vi "lab_3.vi"() -> ()   [LabVIEW 2025]
uses:
  Labview-master/Lab_3/HR_Data_Structure.ctl
  Labview-master/Lab_3/Raw_Data_IN_HR.ctl
  Labview-master/Lab_3/Runner_Data_Structure.ctl
panel:
  out "XY Graph":T1(graph)
  out "BPM":cluster{"Time":timestamp[], "Bpm":i32[]}(graph)
  out "HEART RATE ZONE":string[][](array[string])
  out "error out":errorcluster
  in  "error in":errorcluster
  in  "File Path (dialog if empty)":path
  in  "Runner's Data":T2
  in  "HR Data Structure":T3 {"Raw Data"."Time" format="%<%x %.3X>T"}
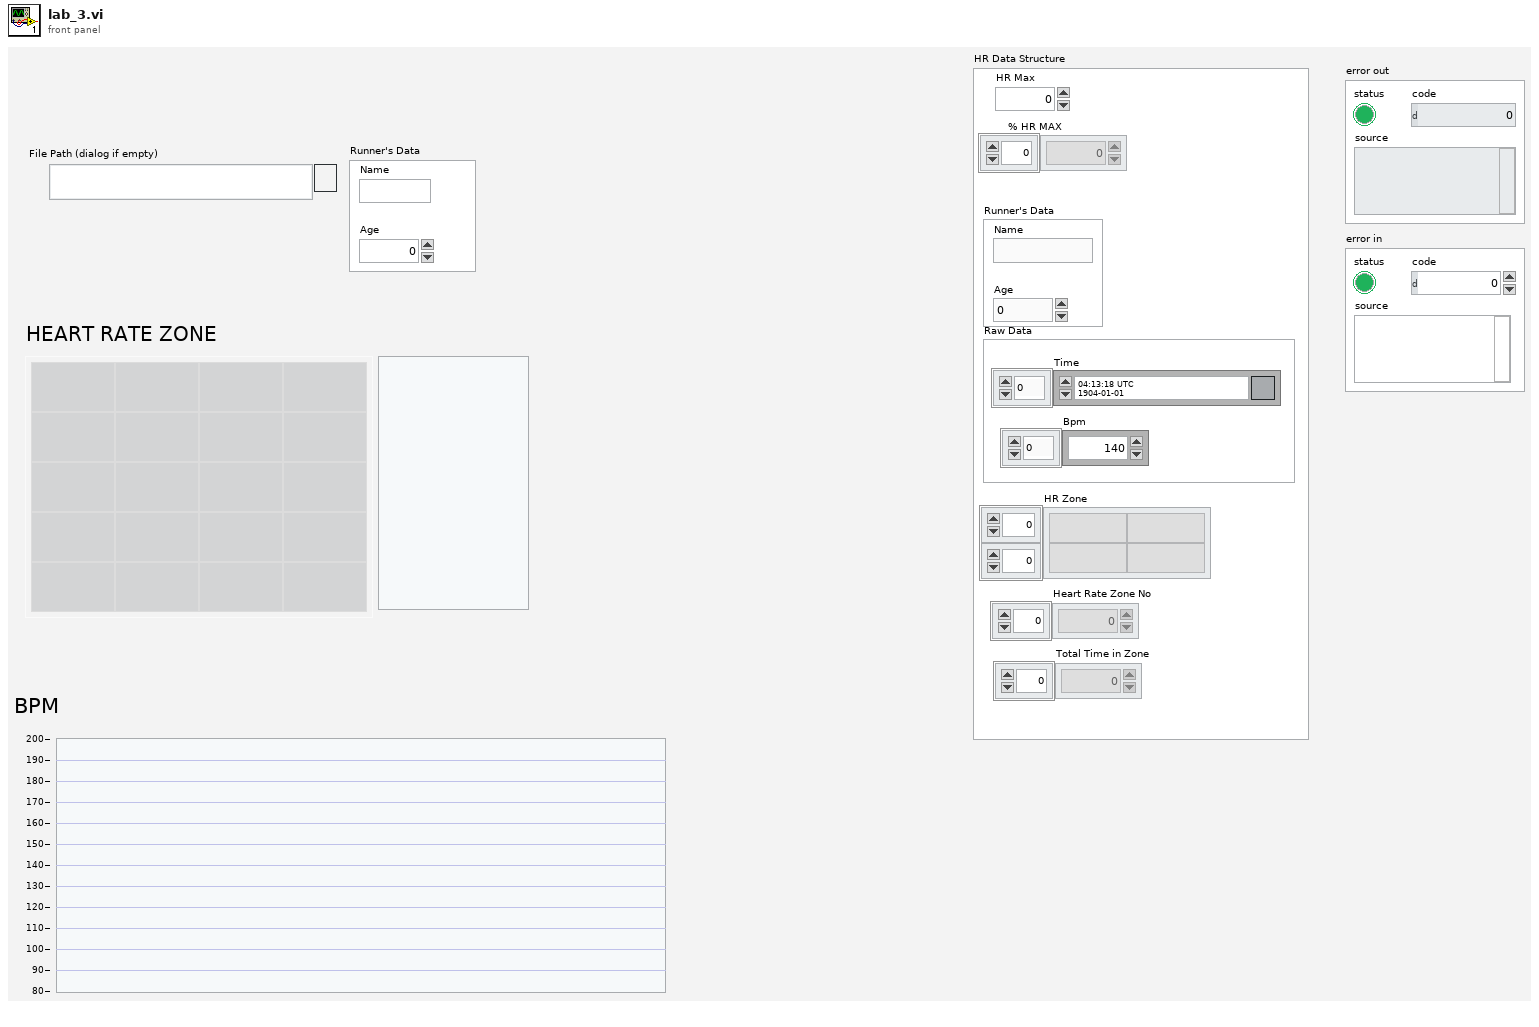
[diagram p1: front panel]
types:
  T1 = cluster{"Total Time in Zone":dbl[], "Heart Rate Zone No":dbl[]}
  T2 = typedef "Runner_Data_Structure.ctl" = cluster{"Name":string, "Age":i32}
  T3 = typedef "HR_Data_Structure.ctl" = cluster{"HR Max":i32, "% HR MAX ":dbl[], "Raw Data":T4, "Runner's Data":T2, "HR Zone":string[][], "Total Time in Zone":dbl[], "Heart Rate Zone No":dbl[]}
  T4 = typedef "Raw_Data_IN_HR.ctl" = cluster{"Time":timestamp[], "Bpm":i32[]}
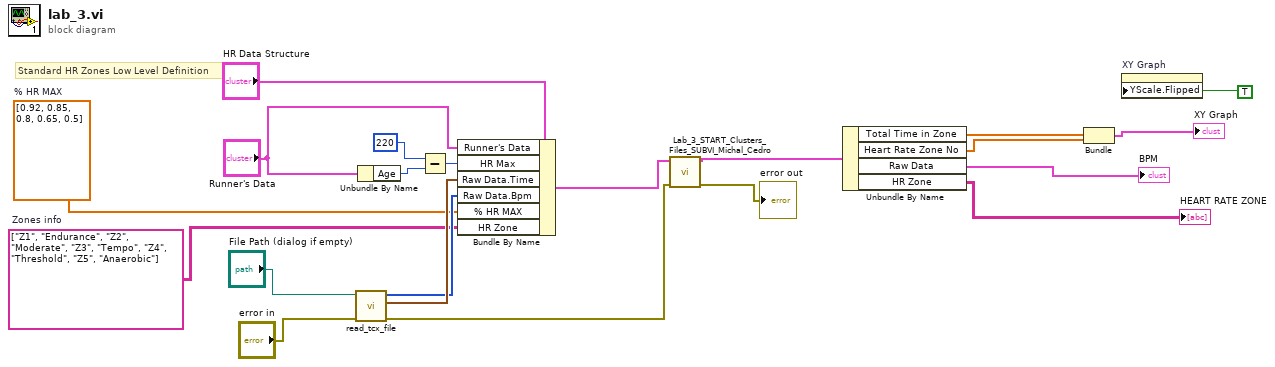
[diagram p0: block diagram]
diagram:
  w8 = string[][] [["Z1", "Endurance"], ["Z2", "Moderate"], ["Z3", "Tempo"], ["Z4", "Threshold"], ["Z5", "Anaerobic"]]  # Zones info
  w9 = dbl[] [0.92, 0.85, 0.8, 0.65, 0.5]  # % HR MAX
  # "Standard HR Zones Low Level Definition"
  n1 = call "read_tcx_file.vi"("error in"="error in", "File Path"="File Path (dialog if empty)") -> ("error out"=w1:errorcluster, "Time"=w14:timestamp[], "Bpm"=w12:i32[])  [unwired: 7 in]
  n2 = Unbundle By Name("Runner's Data") -> ("Age"=w20:i32)
  n3 = Subtract(x=220, y=w20) -> (x-y=w19:i32)
  n4 = Bundle By Name(cluster="HR Data Structure", "Runner's Data"="Runner's Data", "HR Max"=w19, "Raw Data.Time"=w14, "Raw Data.Bpm"=w12, "% HR MAX"=w9, "HR Zone"=w8) -> (w4:T3)
  n5 = call "Lab_3_START_Clusters_Files_SUBVI_Michal_Cedro.vi"("Error IN"=w1, "HR Data Structure IN"=w4) -> ("error out"=→"error out":errorcluster, "HR Data Structure OUT"=w3:T3)  [unwired: 8 in]
  n6 = Unbundle By Name(w3) -> ("Total Time in Zone"=w13:dbl[], "Heart Rate Zone No"=w6:dbl[], "Raw Data"=→"BPM":T4, "HR Zone"=→"HEART RATE ZONE":string[][])
  n7 = Bundle("Total Time in Zone"=w13, "Heart Rate Zone No"=w6) -> (→"XY Graph":T1)  [unwired: 1 in]
  n8 = property on="XY Graph" class="XYGraph (strict)"("YScale.Flipped"=TRUE) -> ()  [unwired: 2 in, 2 out]
